vi "Start Acq.vi"(8 "error in (no error)":errorcluster, 10 "Acquistion Parameters":T1, 11 "Image Acquisition in":refnum<class "Image Acquisition.lvclass">) -> (0 "error out":errorcluster, 3 "Image Acquisition out":refnum<class "Image Acquisition.lvclass">)   [LabVIEW 2016, in "Image Acquisition.lvlib" / "Image Acquisition.lvclass"]
uses:
  Image Acquisition.lvclass
  UI/UI/Controls/Start Acquisition.ctl
  <vilib>/userdefined/High Color/IMAQdx.ctl
  Image Acquisition.lvclass/Image Acquisition.ctl
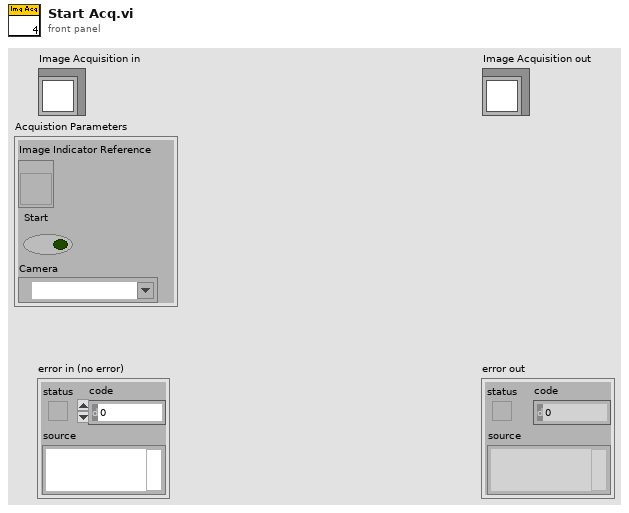
[diagram p1: front panel]
types:
  T1 = typedef "Start Acquisition.ctl" = cluster{"Image Indicator Reference":refnum<vi>, "Start":bool, "Camera":T2}
  T2 = typedef "IMAQdx.ctl" = refnum<k21>
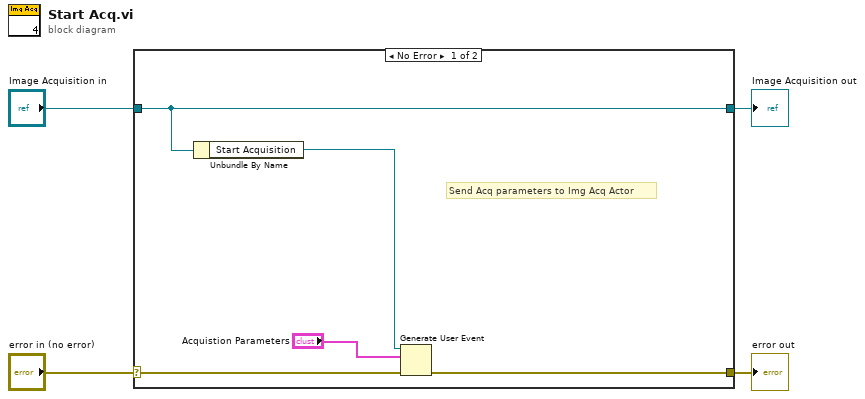
[diagram p0: block diagram]
diagram:
  n1 = case shown="No Error" "error in (no error)" {
    selector: "error in (no error)" -> [w8 w11]
    tunnel: [w7 w11] -> w3
    tunnel: [w9 w10] -> w1
    tunnel: "Image Acquisition in" -> [w9 w10]
    frame No Error {
      # "Send Acq parameters to Img Acq Actor"
      n2 = Unbundle By Name(w9) -> ("Start Acquisition"=w6:refnum<user-event>)
      n3 = Generate User Event(user event=w6, event data cluster="Acquistion Parameters", error in=w8) -> (error out=w7:errorcluster)  [unwired: 1 in, 1 out]
    }
    frame Error {
    }
  }
  "error out" <- w3
  "Image Acquisition out" <- w1
